vi "Arduino_read_wait.vi"() -> ()   [LabVIEW 2015]
uses:
  <vilib>/Instr/_visa.llb/VISA Configure Serial Port (Instr).vi
panel:
  out "String":string
  in  "VISA resource name":refnum<visa-resource-name>
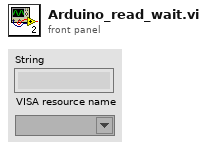
[diagram p1: front panel]
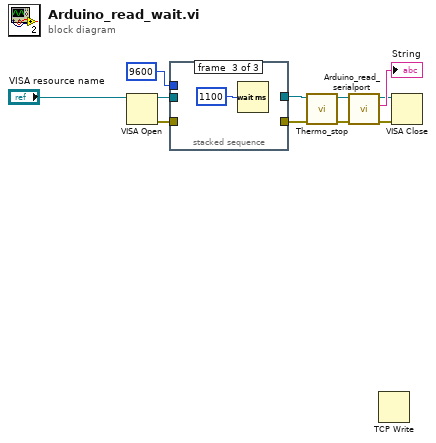
[diagram p0: block diagram]
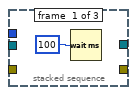
[diagram p2: hidden frame]
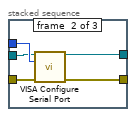
[diagram p3: hidden frame]
diagram:
  n1 = VISA Open(VISA resource name="VISA resource name") -> (VISA resource name=w10:refnum<visa-resource-name>, error out=w9:errorcluster)  [unwired: 4 in]
  n2 = stacked-sequence {
    tunnel: u32 9600 ("baud rate (9600)") -> [_ w17 _]
    tunnel: w10 -> [_ w16 _]
    tunnel: w9 -> [_ w15 _]
    tunnel: [_ w14 _] -> w7
    tunnel: [_ w13 _] -> w6
    frame #0 {
      n3 = Wait (ms)(milliseconds to wait=u32 100) -> ()  [unwired: 1 out]
    }
    frame #1 {
      n4 = call-poly "VISA Configure Serial Port"("VISA resource name"=w16, "baud rate (9600)"=w17, "error in (no error)"=w15) -> ("VISA resource name out"=w14:refnum<visa-resource-name>, "error out"=w13:errorcluster)  [unwired: 11 in]
    }
    frame #2 {
      n5 = Wait (ms)(milliseconds to wait=u32 1100) -> ()  [unwired: 1 out]
    }
  }
  n6 = call "Thermo_stop.vi"("error in (no error)"=w6, "VISA resource name"=w7) -> ("error out"=w4:errorcluster, "VISA resource name out"=w5:refnum<visa-resource-name>)  [unwired: 8 in]
  n7 = call "Arduino_read_serialport.vi"("error in (no error)"=w4, "reference"=w5) -> ("error out"=w2:errorcluster, "String"=→"String":string, "VISA resource name out"=w1:refnum<visa-resource-name>)  [unwired: 6 in, 1 out]
  n8 = TCP Write() -> ()  [unwired: 4 in, 3 out]
  n9 = VISA Close(VISA resource name=w1, error in (no error)=w2) -> ()  [unwired: 1 out]
